vi "SUB-Status string update.vi"(3 "String In":string, 4 "Add Date":bool, 5 "reference":refnum<vi>) -> (2 "String Out":string)   [LabVIEW 2015]
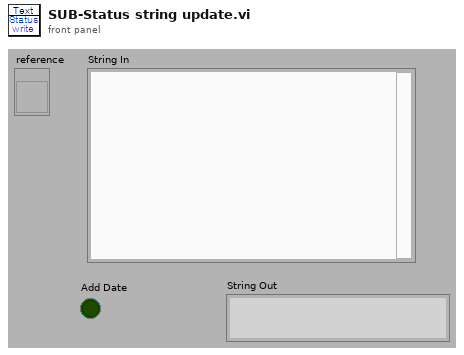
[diagram p1: front panel]
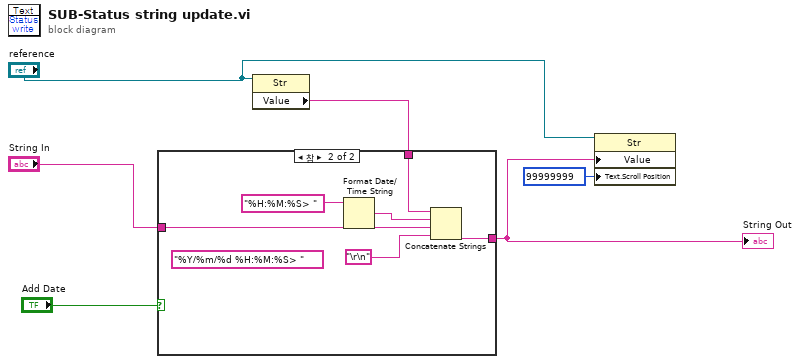
[diagram p0: block diagram]
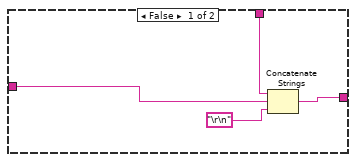
[diagram p2: hidden frame]
diagram:
  n1 = property class="Str"(reference="reference") -> ("Value"=w6:string)  [unwired: 1 in, 2 out]
  n2 = case shown="참" "Add Date" {
    tunnel: w6 -> [w10 w16]
    tunnel: "String In" -> [w8 w13]
    tunnel: [w9 w11] -> w4
    frame False {
      n3 = Concatenate Strings(w10, w8, "\r\n") -> (w9:string)
    }
    frame True {
      (unwired) "%Y/%m/%d %H:%M:%S> " ("상태")
      n4 = Format Date/Time String(time format string (%c)="%H:%M:%S> " ("상태")) -> (date/time string=w14:string)  [unwired: 2 in]
      n5 = Concatenate Strings(w16, w14, w13, "\r\n") -> (w11:string)
    }
  }
  "String Out" <- w4
  n6 = property class="Str"(reference="reference", "Value"=w4, "Text.Scroll Position"=u32 99999999 ("텍스트.스크롤 위치")) -> ()  [unwired: 1 in, 2 out]
